vi "TWS.vi"(0 "System no.":i32=1 min=1 max=4 step=1, 2 "Wavepoint":i32[](array[numeric]), 3 "Trigger value":i32[](array[numeric]), 4 "Switch":i32[](array[numeric]), 5 "error in":errorcluster) -> (14 "Controller error":bool, 19 "error out":errorcluster)   [LabVIEW 2020]
doc: "GCS 1.0: Sets trigger values for point(s) on the waveform and checks for error. Trigger value is bit-mapped. \nGCS 2.0: Defines the trigger state of a certain trigger line for a certain waveform point to high or low.\nController error is TRUE if selected system reports error code not equal to 0. \n\nE-517, E-518: Trigger value is the trigger line to use, can be 1 to 3. Wavepoint can be 1 to 8,192. The power-on default state of all points is low. Afterwards, the signal state of the trigger output line can be switched to \"low\" for all points using the TWC command. It is recommended to use TWC before trigger actions are set with TWS. During the waveform output, the TWS settings will only be used if the configuration of the appropriate trigger line was set with CTO before (set Parameter value \"Generator Trigger\" for CTO Parameter ID \"Trigger Mode\"). During the waveform output, the TWS settings will only be used if the configuration of the appropriate trigger line was set with CTO before (set Parameter value \"Generator Trigger\" for CTO Parameter ID \"Trigger Mode\"). If you start the wave generator with the WGO start options given by bit 3, 4 or 5, the corresponding pulses are output in addition to the output pulses defined with TWS. The number of wave generator output cycles during which trigger pulses are to be output can be set using the Number Of Trigger Cycles parameter, ID 0x18000100. The width of a trigger pulse is 30 µs by default. You can change the default pulse width using the Pulse Width parameter, ID 0x0E000900. Possible values are in the range of 10 to 150 µs.\n\nE-709: Trigger value is the trigger line to use, can be 1 or 2. Line 2 is identical with line 1 here as there is only one trigger table for all wave tables. Wavepoint can be 1 to 16,332. Switch can be 0 (low) or 1 (high). The power-on default state of all points is low. Afterwards, the signal state of the trigger output line can be switched to \"low\" for all points using the TWC command. It is recommended to use TWC before trigger actions are set with TWS. During the waveform output, the TWS settings will only be used if the configuration of the appropriate trigger line was set with CTO before (set Parameter value \"Generator Trigger\" for CTO Parameter ID \"Trigger Mode\"). Only one trigger line per command allowed.\n\nE-710: Wavepoint can be 1-16000. Switch is not valid. Trigger value is bitmapped:\n- Bit 0: trigger line 1: 0 not active, 1 active\n- Bit 1: trigger line 2: 0 not active, 1 active\n- Bit 2: trigger line 3: 0 not active, 1 active\n- Bit 3: trigger line 4: 0 not active, 1 active\n- Bit 8: If = 0, then the Trigger values apply to corresponding Wavepoints only.\nIf = 1, then the Trigger value applies to all points between the last point set by this command and the corresponding Wavepoint point.\n\nE-712: Trigger value is the trigger line to use, can be 1 to 7. Wavepoint can be 1 to 262,144. Switch can be 0 (low) or 1 (high). The power-on default state of all points is low. Afterwards, the signal state of the trigger output line can be switched to \"low\" for all points using the TWC command. It is recommended to use TWC before trigger actions are set with TWS. During the waveform output, the TWS settings will only be used if the configuration of the appropriate trigger line was set with CTO before (set Parameter value \"Generator Trigger\" for CTO Parameter ID \"Trigger Mode\"). Due to the maximum number of parameters per command 10 trigger lines can be set per command call.\n\nE-725: Trigger value is the trigger line to use, can be 1 to 7. Wavepoint can be 1 to 262,144. Switch can be 0 (low) or 1 (high).The power-on default state of all points is low. Afterwards, the signal state of the trigger output line can be switched to \"low\" for all points using the TWC command. It is recommended to use TWC before trigger actions are set with TWS. During the waveform output, the TWS settings will only be used if the configuration of the appropriate trigger line was set with CTO before (set Parameter value \"Generator Trigger\" for CTO Parameter ID \"Trigger Mode\").\n\nE-727: Trigger value is the trigger line to use, can be 1 to 3. Wavepoint can be 1 to 262,144. Switch can be 0 (low) or 1 (high).The power-on default state of all points is low. Afterwards, the signal state of the trigger output line can be switched to \"low\" for all points using the TWC command. It is recommended to use TWC before trigger actions are set with TWS.\n\nE-753: Trigger value is the trigger line to use, can be 1. Wavepoint can be 1 to 65,536. Switch can be 0 (low) or 1 (high). During the waveform output, the TWS settings will only be used if the configuration of the appropriate trigger line was set with CTO before (set Parameter value \"Generator Trigger\" for CTO Parameter ID \"Trigger Mode\").\n\nE-754: Trigger value is the trigger line to use, can be 1. Wavepoint can be 1 to 1,048,576. Switch can be 0 (low) or 1 (high). During the waveform output, the TWS settings will only be used if the configuration of the appropriate trigger line was set with CTO before (set Parameter value \"Generator Trigger\" for CTO Parameter ID \"Trigger Mode\")."
uses:
  Communication.llb/Syntax.ctl
  Communication.llb/Global1.vi
panel:
  # "GCS 1.0: Sets trigger values for point(s) on the waveform and checks for error.\n \"Trigger value\" is bit-mapped.\nGCS 2.0: Defines the trigger state of a certain trigger line for a certain waveform\npoint to high or low."
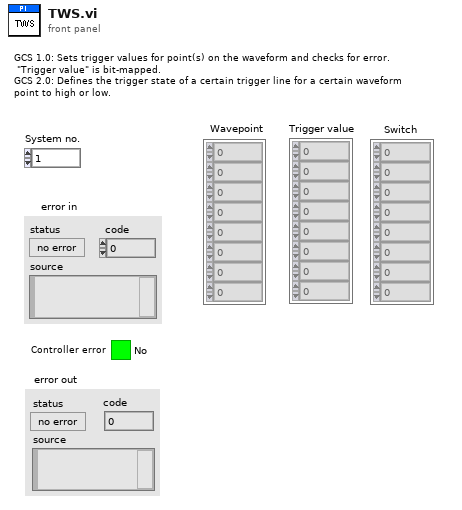
[diagram p1: front panel]
types:
  T1 = typedef "Syntax.ctl" = enum16{"GCS 1.0", "GCS 2.0", "GCS 3.0"}
  T2 = enum16{"Disable error check", "Force error check", "Use global settings"}
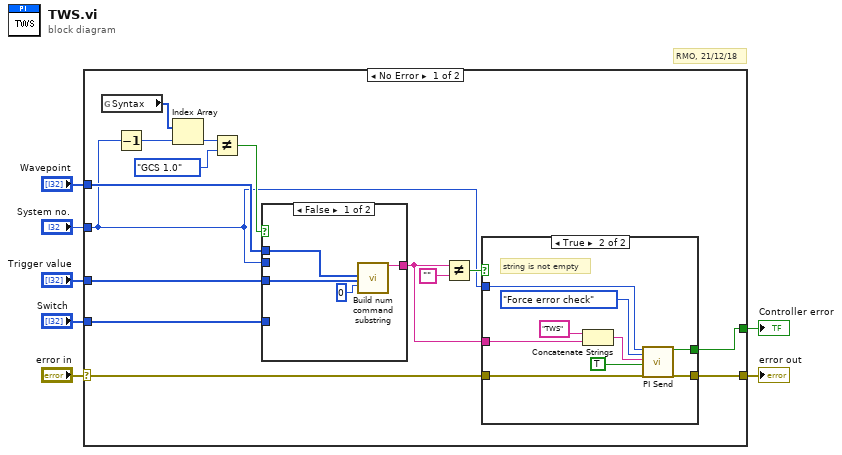
[diagram p0: block diagram]
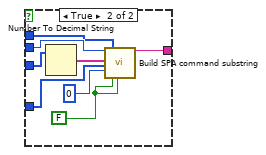
[diagram p2: hidden frame]
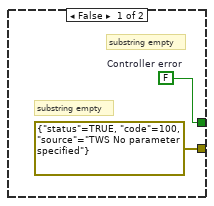
[diagram p3: hidden frame]
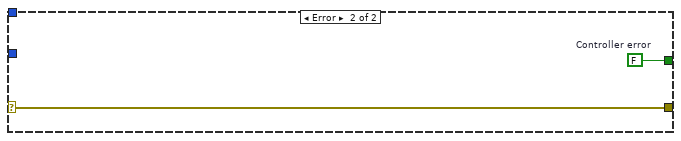
[diagram p4: hidden frame]
diagram:
  # "RMO, 21/12/18"
  n1 = case shown="No Error" "error in" {
    selector: "error in" -> [w10 w47]
    tunnel: [w22 w47] -> w7
    tunnel: "Trigger value" -> [w19 _]
    tunnel: "System no." -> [w12 _]
    tunnel: "Wavepoint" -> [w18 _]
    tunnel: "Switch" -> [w11 _]
    tunnel: [w9 w46] -> w1
    frame No Error {
      n2 = global read "Global1.vi" "Syntax"() -> (w15:T1[])
      n3 = Decrement(x=w12) -> (x-1=w14:i32)
      n4 = Index Array(array=w15, index=w14) -> (element=w16:T1)
      n5 = Not Equal?(x=w16, y=Syntax."GCS 1.0") -> (x != y?=w13:bool)
      n6 = case shown="False" w13 {
        tunnel: [w26 w30] -> w20
        tunnel: w19 -> [w25 w28]
        tunnel: w18 -> [w24 w27]
        tunnel: w12 -> [_ w34]
        tunnel: w11 -> [_ w31]
        frame False {
          n7 = call "Build num command substring.vi"("Num 1"=w24, "Num 2"=w25, "No. of digits"=i16 0) -> ("Command substring"=w26:string)  [unwired: 16 out]
        }
        frame True {
          w32 = FALSE ("Parameter no. format \n(Decimal: FALSE)")
          n8 = Number To Decimal String(number=w28) -> (decimal integer string=w33:string[])  [unwired: 1 out]
          n9 = call "Build SPA command substring.vi"("System no."=w34, "Axes to set"=w33, "Parameter values"=w31, "No. of digits"=i16 0, "Parameter number"=w27, "Parameter no. format \n(Decimal: FALSE)"=w32, "Parameter format \n(Num.: FALSE)"=w32) -> ("SPA command substring"=w30:string)  [unwired: 3 in, 9 out]
        }
      }
      n10 = Not Equal?(x=w20, y="") -> (x != y?=w17:bool)
      n11 = case shown="True" w17 {
        tunnel: w20 -> [_ w44]
        tunnel: [errorcluster {"status"=TRUE, "code"=100, "source"="TWS No parameter specified"} ("error out") w38] -> w22
        tunnel: w10 -> [_ w41]
        tunnel: w12 -> [_ w40]
        tunnel: [w35 w37] -> w9
        frame False {
          w35 = FALSE  # Controller error
          # "substring empty"
          # "substring empty"
        }
        frame True {
          # "string is not empty"
          n12 = Concatenate Strings("TWS", w44) -> (w42:string)
          n13 = call "PI Send.vi"("System no."=w40, "Error check settings"=T2."Force error check", "String to send"=w42, "Attach termination char.?"=TRUE ("Attach Linefeed?"), "error in"=w41) -> ("Controller error"=w37:bool, "error out"=w38:errorcluster)  [unwired: 1 in, 12 out]
        }
      }
    }
    frame Error {
      w46 = FALSE  # Controller error
    }
  }
  "error out" <- w7
  "Controller error" <- w1
